vi "Page_Advanced_Write.vi"(6 "ctlReferences":T1, 8 "error in (no error)":errorcluster, 11 "Class in":refnum<class "IB_MSI.lvclass">) -> (0 "error out":errorcluster, 3 "Class out":refnum<class "IB_MSI.lvclass">)   [LabVIEW 2020, in "IB_MSI.lvclass"]
uses:
  <vilib>/AppBuilder/IB_Classes/MSI/IB_MSI.lvclass
  <vilib>/AppBuilder/IB_Classes/MSI/IB_MSI.lvclass/IB_MSI.ctl
  <vilib>/AppBuilder/IB_Classes/Installer/Installer.lvclass
  <resource>/Framework/Providers/Builds/Installer/Pages/controls/IB_UI_Page_Advanced_References.ctl
  <resource>/Framework/Providers/Builds/Installer/CDK_sTypeDef_SystemRequirements.ctl
  <resource>/Framework/Providers/Common/provcom_BrowseProjectFile2.ctl
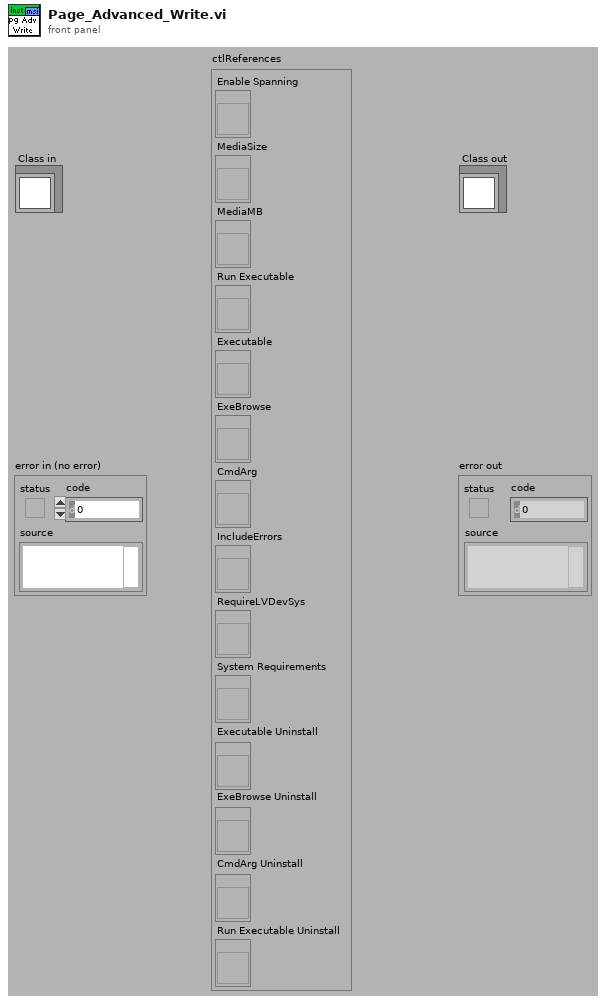
[diagram p1: front panel]
types:
  T1 = typedef "IB_UI_Page_Advanced_References.ctl" = cluster{"Enable Spanning":refnum<vi>, "MediaSize":refnum<vi>, "MediaMB":refnum<vi>, "Run Executable":refnum<vi>, "Executable":refnum<vi>, "ExeBrowse":refnum<vi>, "CmdArg":refnum<vi>, "IncludeErrors":refnum<vi>, "RequireLVDevSys":refnum<vi>, "System Requirements":refnum<vi>, "Executable Uninstall":refnum<vi>, "ExeBrowse Uninstall":refnum<vi>, "CmdArg Uninstall":refnum<vi>, "Run Executable Uninstall":refnum<vi>}
  T2 = typedef "CDK_sTypeDef_SystemRequirements.ctl" = u16
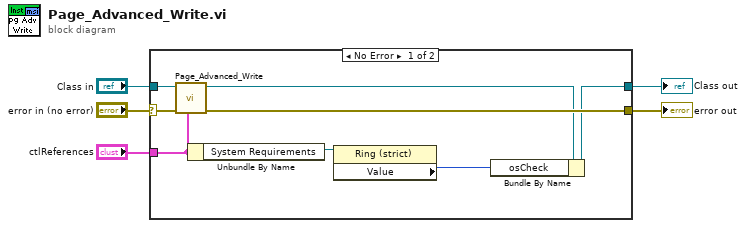
[diagram p0: block diagram]
diagram:
  n1 = case shown="No Error" "error in (no error)" {
    selector: "error in (no error)" -> [w11 w15]
    tunnel: [w10 w15] -> w4
    tunnel: [w7 w14] -> w2
    tunnel: "Class in" -> [w12 w14]
    tunnel: "ctlReferences" -> [w9 _]
    frame No Error {
      n2 = call-parent "Page_Advanced_Write.vi"("ctlReferences"=w9, "error in (no error)"=w11, "Class in"=w12) -> ("error out"=w10:errorcluster, "Class out"=w8:refnum<class "IB_MSI.lvclass">)  [unwired: 7 out]
      n3 = Unbundle By Name(w9) -> ("System Requirements"=w13:refnum<vi>)
      n4 = property class="Ring (strict)"(reference=w13) -> ("Value"=w6:T2)  [unwired: 1 in, 2 out]
      n5 = Bundle By Name(cluster=w8, "osCheck"=w6) -> (w7:refnum<class "IB_MSI.lvclass">)
    }
    frame Error {
    }
  }
  "error out" <- w4
  "Class out" <- w2
